vi "Install Runtime Engine 2012 NIVerified.vi"(5 "Files Generated by Build":path[](array[path]), 6 "Top Level/Always Included VIs":path[](array[path]), 7 "Destination Path":path, 8 "error in (no error)":errorcluster, 9 "Target Name":string, 10 "Build Specification Name":string, 11 "Project Path":path) -> (0 "error out":errorcluster)   [LabVIEW 2022 SP3]
doc: "This VI is intended to be used as a Post Build Action in a Build Application Specification on Mac. The VI installs the LabVIEW Run-Time Engine inside the built application so that it can be used as a completely standalone application and not depend on a separate installation of the LabVIEW Run-Time Engine."
panel:
  # "Overview: This VI is intended to be used as a Post Build Action in a Build Application Specification on Mac. The VI installs the LabVIEW Run-Time Engine inside the built application\nRequirements: LabVIEW 2012 (or compatible), Mac with OS X\nInstructions:\n1. Create a new project\n2. Create a build specification  \n3. Set this VI as the \"Execute VI after build\"\n4. Build the project"
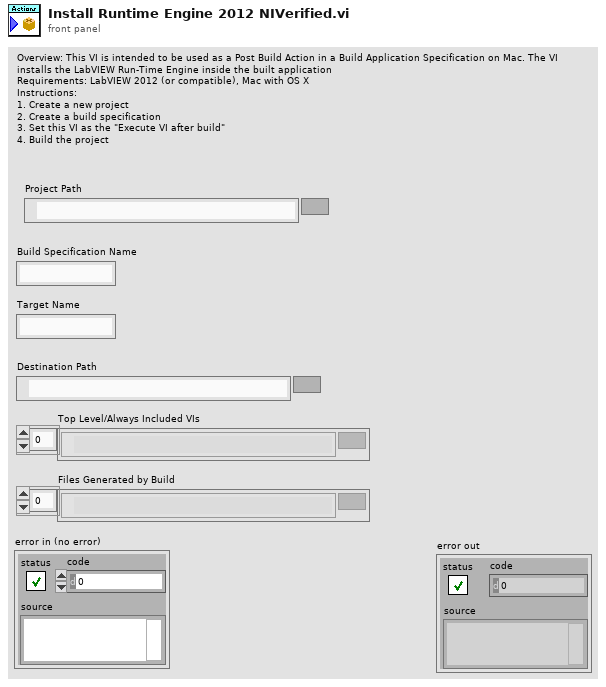
[diagram p1: front panel]
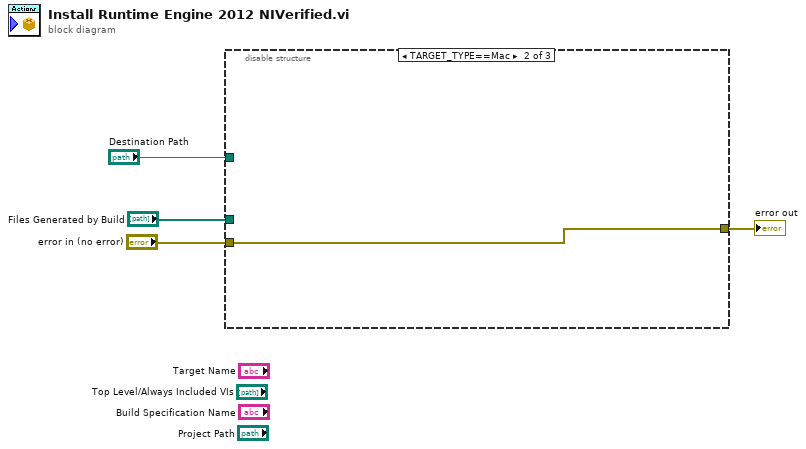
[diagram p0: block diagram]
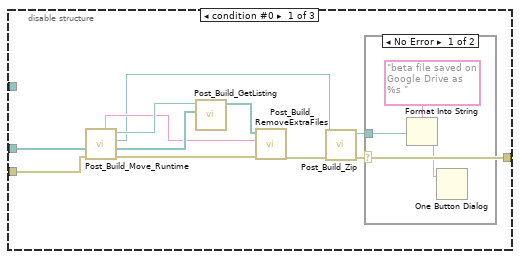
[diagram p2: hidden frame]
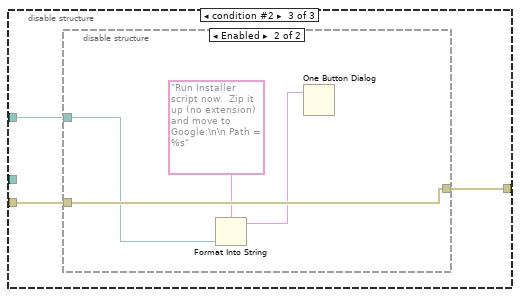
[diagram p4: hidden frame]
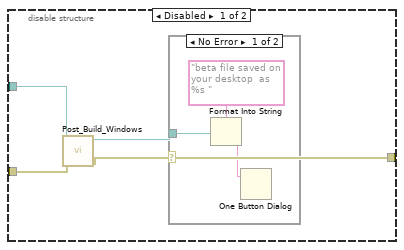
[diagram p5: hidden frame]
diagram:
  n1 = disable-structure shown="TARGET_TYPE==Mac" {
    disable-tunnel: "Files Generated by Build" -> [w9 _ _]
    disable-tunnel: "error in (no error)" -> [w8 w19 w21]
    disable-tunnel: [w7 w19 w20] -> w2
    disable-tunnel: "Destination Path" -> [_ _ w22]
    frame condition #0 {
      n2 = call "Post_Build_Move_Runtime.vi"("error in (no error)"=w8, "Files in"=w9) -> ("error out"=w12:errorcluster, "Files out"=w14:path[], "Path"=w6:path, "Runtime Path"=w15:path, "LV Version"=w11:string)  [unwired: 5 in]
      n3 = call "Post_Build_GetListing.vi"("Files Generated by Build"=w14, "Runtime Path"=w15) -> ("Files to clear"=w13:path[])  [unwired: 9 in]
      n4 = call "Post_Build_RemoveExtraFiles.vi"("error in (no error)"=w12, "Rumtime Name"=w11, "Files to remove"=w13) -> ("error out"=w10:errorcluster)  [unwired: 8 in]
      n5 = call "Post_Build_Zip.vi"("error in (no error)"=w10, "Path"=w6) -> ("error out"=w7:errorcluster, "Zip File"=w5:path)  [unwired: 8 in]
      n6 = case shown="No Error" w7 {
        tunnel: w5 -> [w16 _]
        frame No Error {
          n7 = Format Into String(format string="beta file saved on Google Drive as %s " ("message"), w16) -> (resulting string=w17:string)  [unwired: 2 in, 1 out]
          n8 = One Button Dialog(message=w17) -> ()  [unwired: 1 in, 1 out]
        }
        frame Error {
        }
      }
    }
    frame condition #1 (active) {
    }
    frame condition #2 {
      n9 = disable-structure shown="Enabled" {
        disable-tunnel: w22 -> [w26 w32]
        disable-tunnel: w21 -> [w25 w33]
        disable-tunnel: [w24 w33] -> w20
        frame Disabled {
          n10 = call "Post_Build_Windows.vi"("error in (no error)"=w25, "Destination Path"=w26) -> ("error out"=w24:errorcluster, "Zip File"=w23:path)  [unwired: 8 in]
          n11 = case shown="No Error" w24 {
            tunnel: w23 -> [w27 _]
            frame No Error {
              n12 = Format Into String(format string="beta file saved on your desktop  as %s " ("message"), w27) -> (resulting string=w28:string)  [unwired: 2 in, 1 out]
              n13 = One Button Dialog(message=w28) -> ()  [unwired: 1 in, 1 out]
            }
            frame Error {
            }
          }
        }
        frame Enabled {
          n14 = Format Into String(format string="Run Installer script now.  Zip it up (no extension) and move to Google:\n\n Path = %s" ("message"), w32) -> (resulting string=w31:string)  [unwired: 2 in, 1 out]
          n15 = One Button Dialog(message=w31) -> ()  [unwired: 1 in, 1 out]
        }
      }
    }
  }
  "error out" <- w2
